vi "rx queue.vi"(8 "error in (no error)":errorcluster, 11 "data passing":T1) -> (0 "error out":errorcluster, 3 "data passing out":T1)   [LabVIEW 2016]
uses:
  data.ctl
  device/device.ctl
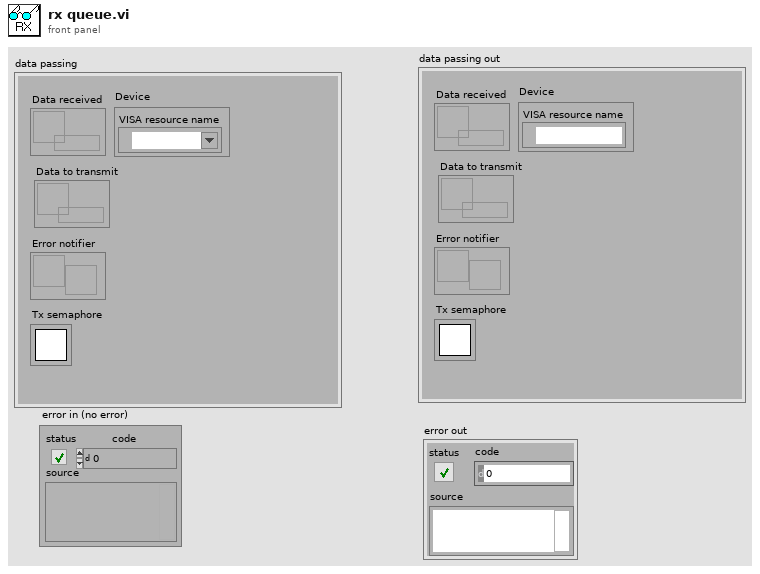
[diagram p1: front panel]
types:
  T1 = typedef "data.ctl" = cluster{"Data received":refnum<queue>, "Data to transmit":refnum<queue>, "Error notifier":refnum<notifier>, "Tx semaphore":T2, "Device":T3}
  T2 = typedef "Semaphore RefNum" = refnum<k1>
  T3 = typedef "device.ctl" = cluster{"VISA resource name":refnum<visa-resource-name>}
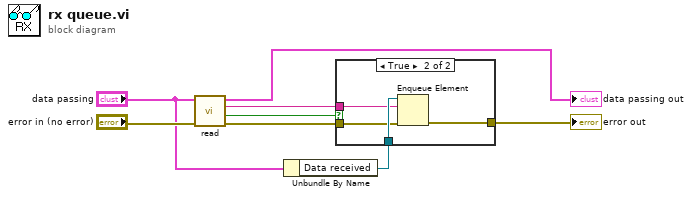
[diagram p0: block diagram]
diagram:
  n1 = call "read.vi"("error in (no error)"="error in (no error)", "data passing"="data passing") -> ("error out"=w5:errorcluster, "full command?"=w4:bool, "packet"=w1:string, "data passing out"=→"data passing out":T1)  [unwired: 6 in]
  n2 = Unbundle By Name("data passing") -> ("Data received"=w7:refnum<queue>)
  n3 = case shown="True" w4 {
    tunnel: [w9 w13] -> w8
    tunnel: w7 -> [_ w12]
    tunnel: w5 -> [w9 w11]
    tunnel: w1 -> [_ w10]
    frame False {
    }
    frame True {
      n4 = Enqueue Element(queue=w12, element=w10, error in (no error)=w11) -> (error out=w13:errorcluster)  [unwired: 1 in, 2 out]
    }
  }
  "error out" <- w8
